vi "Histogram Main.vi"() -> ()   [LabVIEW 2012]
uses:
  Consumer Message.ctl
  <vilib>/Utility/file.llb/Write To Spreadsheet File (DBL).vi
panel:
  in  "信号":u16(ring) items=["均匀白噪声", "均匀+均匀", "高斯白噪声", "正弦波", "方波"]
  in  "快照":bool
  out "直方图":cluster{"histogram":dbl[], "x axis":dbl[]}(graph)
  in  "区间":i32=20
  out "消费者关闭？":bool
  out "积压空间":u8(slide) scale=0.0..100.0
  in  "停止":bool
  # "待入队处理的消息数量"
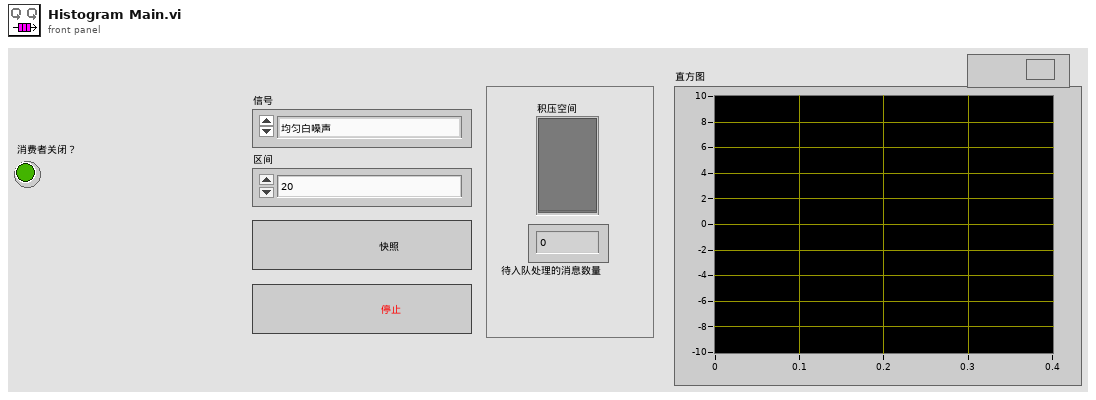
[diagram p1: front panel]
types:
  T1 = typedef "Consumer Message.ctl" = cluster{"消费者状态":string, "布尔数据":bool, "数值数据":i32, "信号":dbl[], "错误":cluster{"状态":bool, "代码":i32, "源":string}}
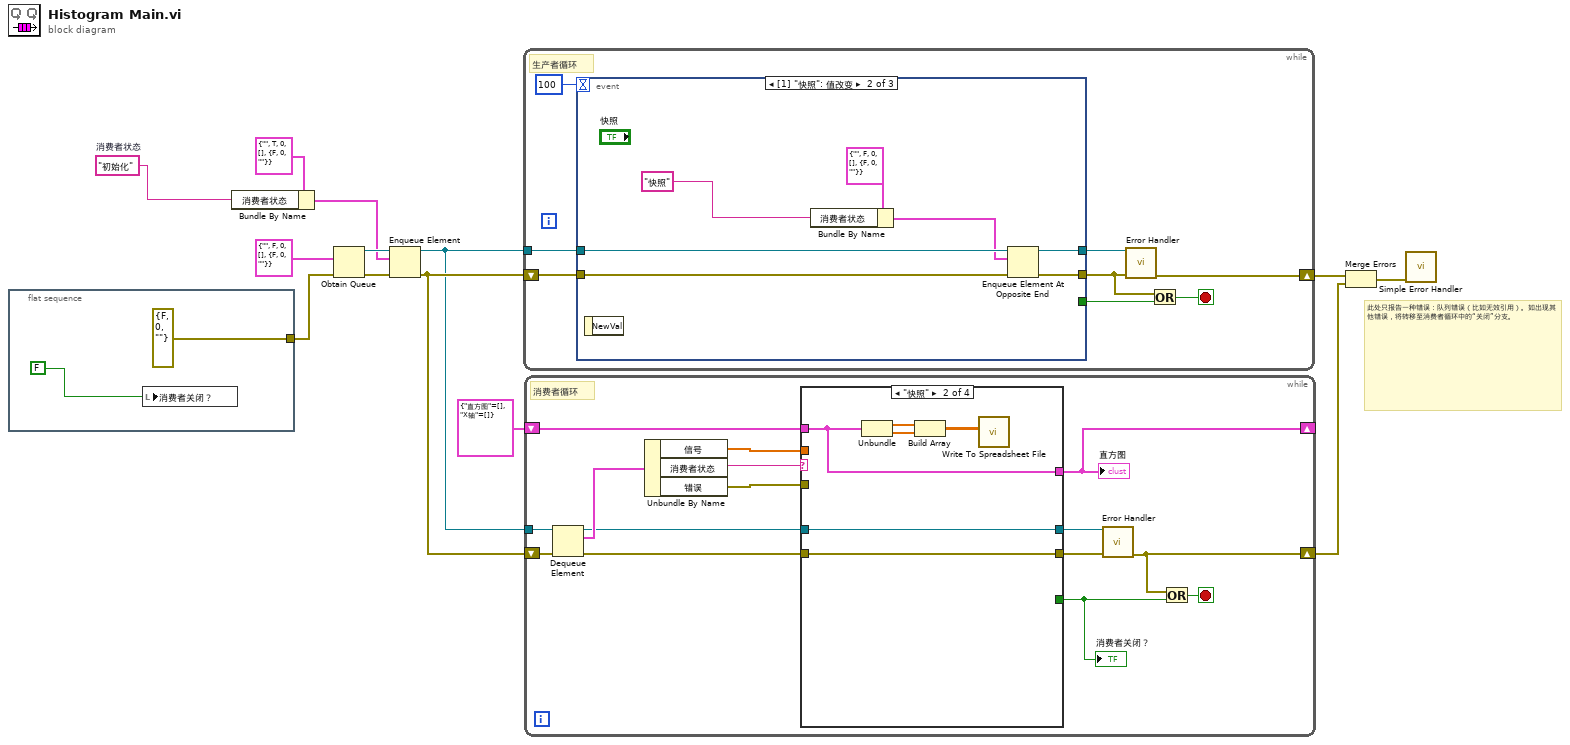
[diagram p0: block diagram]
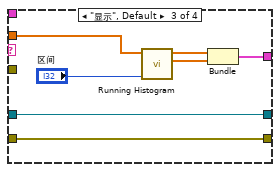
[diagram p3: hidden frame]
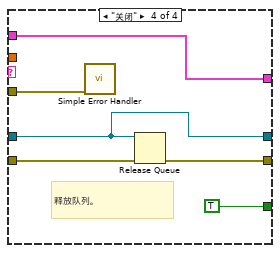
[diagram p4: hidden frame]
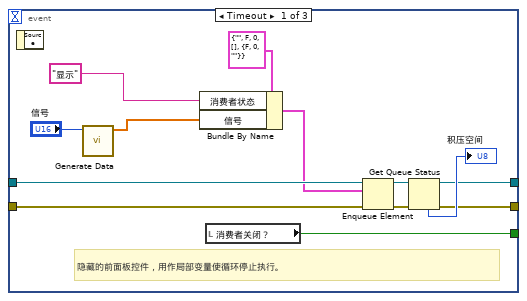
[diagram p5: hidden frame]
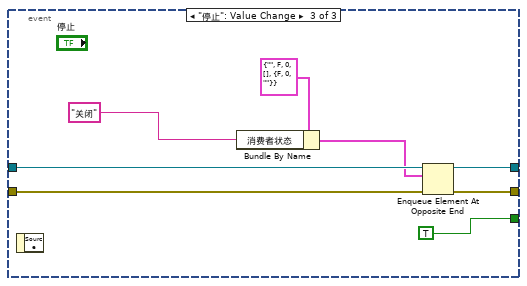
[diagram p6: hidden frame]
diagram:
  w5 = "初始化"  # 消费者状态
  # "此处只报告一种错误：队列错误（比如无效引用）。如出现其他错误，将转移至消费者循环中的“关闭”分支。"
  n1 = flat-sequence {
    tunnel: [cluster{"状态":bool, "代码":i32, "源":string} {"状态"=FALSE, "代码"=0, "源"=""} ("错误输入（无错误）")] -> w8
    frame #0 {
      n2 = local write "消费者关闭？"(FALSE ("停止循环（局部）")) -> ()
    }
  }
  n3 = Bundle By Name ("按名称捆绑")(cluster=T1 {"消费者状态"="", "布尔数据"=TRUE, "数值数据"=0, "信号"=[], "错误"={"状态"=FALSE, "代码"=0, "源"=""}} ("消费者消息"), "消费者状态"=w5) -> (w6:T1)
  n4 = Obtain Queue ("获取队列引用")(element data type=T1 {"消费者状态"="", "布尔数据"=FALSE, "数值数据"=0, "信号"=[], "错误"={"状态"=FALSE, "代码"=0, "源"=""}}, error in (no error)=w8) -> (queue out=w10:refnum<queue>, error out=w13:errorcluster)  [unwired: 3 in, 1 out]
  n5 = Enqueue Element ("元素入队列")(queue=w10, element=w6, error in (no error)=w13) -> (queue out=w9:refnum<queue>, error out=w11:errorcluster)  [unwired: 1 in, 1 out]
  n6 = while {
    tunnel: w9 -> [w23]
    shift-right: [w16] -> w4
    shift-left: w11 -> [w22]
    stop <- w18 stop-if-true
    # "生产者循环"
    n7 = event shown="[1] \"快照\": 值改变" {
      selector: _ -> [_ _ _]
      dyn-events: _ -> [_ _ _]
      timeout: 100 -> [_ _ _]
      tunnel: w23 -> [w34 w42 w51]
      tunnel: w22 -> [w30 w41 w49]
      tunnel: [w33 w43 w48] -> w17
      tunnel: [w36 _ TRUE] -> w19
      tunnel: [w32 w38 w47] -> w21
      event Timeout {
        # "隐藏的前面板控件，用作局部变量使循环停止执行。"
        n8 = event-data ("事件数据节点")() -> ()  [unwired: 1 in, 1 out]
        n9 = call "Generate Data.vi"("信号"="信号") -> ("Y"=w26:dbl[])  [unwired: 9 in, 1 out]
        n10 = Bundle By Name ("按名称捆绑")(cluster=T1 {"消费者状态"="", "布尔数据"=FALSE, "数值数据"=0, "信号"=[], "错误"={"状态"=FALSE, "代码"=0, "源"=""}}, "消费者状态"="显示", "信号"=w26) -> (w27:T1)
        n11 = local read "消费者关闭？"() -> (w36:bool)
        n12 = Enqueue Element ("元素入队列")(queue=w34, element=w27, error in (no error)=w30) -> (queue out=w31:refnum<queue>, error out=w29:errorcluster)  [unwired: 1 in, 1 out]
        n13 = Get Queue Status ("获取队列状态")(queue=w31, error in (no error)=w29) -> (queue out=w32:refnum<queue>, error out=w33:errorcluster, # elements in queue=→"积压空间":i32)  [unwired: 1 in, 5 out]
      }
      event "快照": Value Change {
        n14 = event-data ("事件数据节点")() -> ()  [unwired: 1 in, 1 out]
        n15 = Bundle By Name ("按名称捆绑")(cluster=T1 {"消费者状态"="", "布尔数据"=FALSE, "数值数据"=0, "信号"=[], "错误"={"状态"=FALSE, "代码"=0, "源"=""}}, "消费者状态"="快照" ("字符串数据")) -> (w39:T1)
        n16 = Enqueue Element At Opposite End ("队列最前端插入元素")(queue=w42, element=w39, error in (no error)=w41) -> (queue out=w38:refnum<queue>, error out=w43:errorcluster)  [unwired: 1 in, 1 out]
      }
      event "停止": Value Change {
        n17 = event-data ("事件数据节点")() -> ()  [unwired: 1 in, 1 out]
        n18 = Bundle By Name ("按名称捆绑")(cluster=T1 {"消费者状态"="", "布尔数据"=FALSE, "数值数据"=0, "信号"=[], "错误"={"状态"=FALSE, "代码"=0, "源"=""}}, "消费者状态"="关闭") -> (w44:T1)
        n19 = Enqueue Element At Opposite End ("队列最前端插入元素")(queue=w51, element=w44, error in (no error)=w49) -> (queue out=w47:refnum<queue>, error out=w48:errorcluster)  [unwired: 1 in, 1 out]
      }
    }
    n20 = call "Error Handler.vi"("错误输入"=w17, "队列输入"=w21) -> ("错误输出"=w16:cluster{"状态":bool, "代码":i32, "源":string})  [unwired: 8 in, 1 out]
    n21 = Or ("或")(x=w17, y=w19) -> (x .or. y?=w18:bool)
  }
  n22 = while {
    tunnel: w9 -> [w66]
    shift-right: [w57] -> w3
    shift-left: w11 -> [w65]
    shift-right: [w54] -> _
    shift-left: cluster{"直方图":dbl[], "X轴":dbl[]} {"直方图"=[], "X轴"=[]} -> [w53]
    stop <- w58 stop-if-true
    # "消费者循环"
    n23 = Dequeue Element ("元素出队列")(queue=w66, error in (no error)=w65) -> (queue out=w56:refnum<queue>, element=w64:T1, error out=w55:errorcluster)  [unwired: 1 in, 1 out]
    n24 = Unbundle By Name ("按名称解除捆绑")(w64) -> ("信号"=w52:dbl[], "消费者状态"=w63:string, "错误"=w60:cluster{"状态":bool, "代码":i32, "源":string})
    n25 = case shown="\"快照\"" w63 {
      tunnel: [_ _ _ TRUE] -> w59
      tunnel: w55 -> [w68 w74 w81 w87]
      tunnel: [w68 w74 w81 w86] -> w62
      tunnel: w56 -> [w69 w75 w82 w84]
      tunnel: [w69 w75 w82 w84] -> w61
      tunnel: w60 -> [_ _ _ w85]
      tunnel: [w67 w70 w77 w83] -> w54
      tunnel: w53 -> [w67 w70 _ w83]
      tunnel: w52 -> [_ _ w76 _]
      frame "初始化" {
      }
      frame "快照" {
        n26 = Unbundle ("解除捆绑")(w70) -> ("直方图"=w73:dbl[], "X轴"=w72:dbl[])
        n27 = Build Array ("创建数组")(w73, w72) -> (w71:dbl[][])
        n28 = call-poly <vilib>:"Write To Spreadsheet File.vi"("2D data"=w71) -> ()  [unwired: 7 in, 1 out]
      }
      frame "显示", Default {
        n29 = call "Running Histogram.vi"("区间"="区间", "输入数据"=w76) -> ("X轴"=w78:dbl[], "直方图"=w79:dbl[])  [unwired: 6 in, 2 out]
        n30 = Bundle ("捆绑")("直方图"=w79, "X轴"=w78) -> (w77:cluster{"直方图":dbl[], "X轴":dbl[]})  [unwired: 1 in]
      }
      frame "关闭" {
        # "释放队列。"
        n31 = call <vilib>:"Simple Error Handler.vi"("error in (no error)"=w85) -> ()  [unwired: 4 in, 5 out]
        n32 = Release Queue ("释放队列引用")(queue=w84, error in (no error)=w87) -> (error out=w86:errorcluster)  [unwired: 1 in, 2 out]
      }
    }
    "消费者关闭？" <- w59
    "直方图" <- w54
    n33 = call "Error Handler.vi"("错误输入"=w62, "队列输入"=w61) -> ("错误输出"=w57:cluster{"状态":bool, "代码":i32, "源":string})  [unwired: 8 in, 1 out]
    n34 = Or ("或")(x=w57, y=w59) -> (x .or. y?=w58:bool)
  }
  n35 = Merge Errors ("合并错误")(w4, w3) -> (w2:errorcluster)
  n36 = call <vilib>:"Simple Error Handler.vi"("error in (no error)"=w2) -> ()  [unwired: 4 in, 5 out]
